vi "Write ADC Type.vi"(8 "error in (no error)":errorcluster, 10 "ADC Type":T1, 11 "LINX-ADS1X15 in":refnum<class "LINX-ADS1256.lvclass">) -> (0 "error out":errorcluster, 3 "LINX-ADS1X15 out":refnum<class "LINX-ADS1256.lvclass">)   [LabVIEW 2020]
uses:
  LINX-ADS1256.lvclass
  ADC Type Selection.ctl
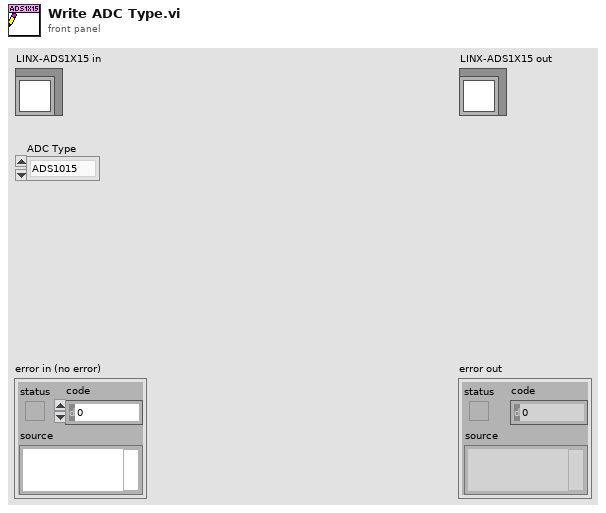
[diagram p1: front panel]
types:
  T1 = typedef "LINX-ADS1256.lvclass/ADC Type Selection.ctl" = enum16{"ADS1015", "ADS1115"}
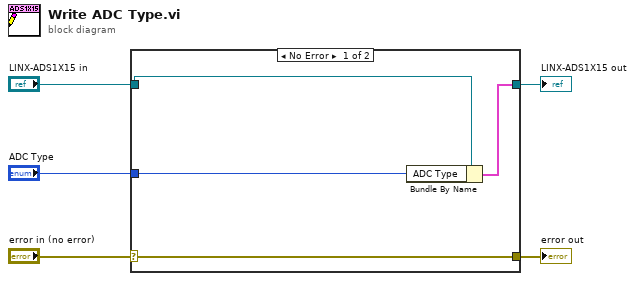
[diagram p0: block diagram]
diagram:
  n1 = case shown="No Error" "error in (no error)" {
    selector: "error in (no error)" -> [w9 w10]
    tunnel: [w9 w10] -> w4
    tunnel: [w7 w11] -> w2
    tunnel: "LINX-ADS1X15 in" -> [w8 w11]
    tunnel: "ADC Type" -> [w6 _]
    frame No Error {
      n2 = Bundle By Name(cluster=w8, "ADC Type"=w6) -> (w7:cluster{})
    }
    frame Error {
    }
  }
  "error out" <- w4
  "LINX-ADS1X15 out" <- w2
